vi "LABVIEWWIPPROJECT.vi"() -> ()   [LabVIEW 2025]
panel:
  out "Balance":dbl
  out "Jackpot":bool
  out "minor prize":bool
  out "String":string
  in  "Bet amount":i32
  out "Array of Nums":dbl[](array[numeric])
  out "Major Prize":bool
  in  "SPIN":bool
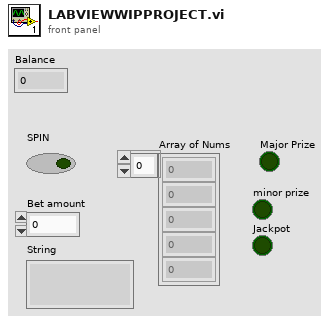
[diagram p1: front panel]
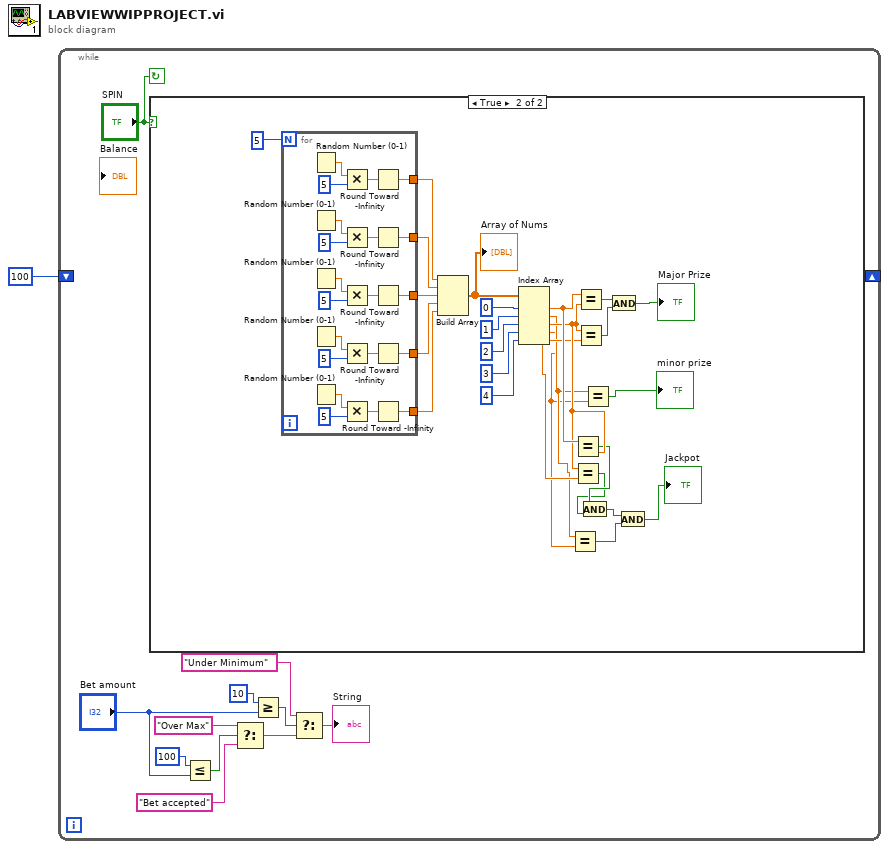
[diagram p0: block diagram]
diagram:
  n1 = while {
    shift-right: _ -> [_]
    shift-left: 100 -> [_]
    stop <- "SPIN" continue-if-true
    n2 = case shown="True" "SPIN" {
      frame False {
      }
      frame True {
        n3 = for {
          N: 5 -> [_]
          tunnel: [w43] -> w30
          tunnel: [w42] -> w29
          tunnel: [w41] -> w28
          tunnel: [w40] -> w27
          tunnel: [w39] -> w26
          n4 = Random Number (0-1)() -> (number: 0 to 1=w58:dbl)
          n5 = Random Number (0-1)() -> (number: 0 to 1=w55:dbl)
          n6 = Random Number (0-1)() -> (number: 0 to 1=w52:dbl)
          n7 = Random Number (0-1)() -> (number: 0 to 1=w49:dbl)
          n8 = Random Number (0-1)() -> (number: 0 to 1=w46:dbl)
          n9 = Multiply(x=w58, y=5) -> (x*y=w56:dbl)
          n10 = Multiply(x=w55, y=5) -> (x*y=w53:dbl)
          n11 = Multiply(x=w52, y=5) -> (x*y=w50:dbl)
          n12 = Multiply(x=w49, y=5) -> (x*y=w47:dbl)
          n13 = Multiply(x=w46, y=5) -> (x*y=w44:dbl)
          n14 = Round Toward -Infinity(1:w56) -> (0:w43:dbl)
          n15 = Round Toward -Infinity(1:w53) -> (0:w42:dbl)
          n16 = Round Toward -Infinity(1:w50) -> (0:w41:dbl)
          n17 = Round Toward -Infinity(1:w47) -> (0:w40:dbl)
          n18 = Round Toward -Infinity(1:w44) -> (0:w39:dbl)
        }
        n19 = Build Array(w30, w29, w28, w27, w26) -> (w25:dbl[])
        "Array of Nums" <- w25
        n20 = Index Array(array=w25, index #1=0, index #2=1, index #3=2, index #4=3, index #5=4) -> (element #1=w22:dbl, element #2=w19:dbl, element #3=w21:dbl, element #4=w18:dbl, element #5=w20:dbl)
        n21 = Equal?(x=w19, y=w18) -> (x = y?=w14:bool)
        n22 = Equal?(x=w22, y=w21) -> (x = y?=w17:bool)
        n23 = Equal?(x=w21, y=w20) -> (x = y?=w16:bool)
        n24 = Equal?(x=w22, y=w21) -> (x = y?=w37:bool)
        n25 = Equal?(x=w21, y=w20) -> (x = y?=w31:bool)
        n26 = And(x=w17, y=w16) -> (x .and. y?=w15:bool)
        n27 = Equal?(x=w19, y=w18) -> (x = y?=→"minor prize":bool)
        n28 = And(x=w37, y=w31) -> (x .and. y?=→"Major Prize":bool)
        n29 = And(x=w15, y=w14) -> (x .and. y?=→"Jackpot":bool)
      }
    }
    n30 = Less Or Equal?(x=100, y="Bet amount") -> (x <= y?=w6:bool)
    n31 = Select(t="Over Max", s=w6, f="Bet accepted") -> (s? t:f=w3:string)
    n32 = Greater Or Equal?(x=10, y="Bet amount") -> (x >= y?=w5:bool)
    n33 = Select(t="Under Minimum", s=w5, f=w3) -> (s? t:f=→"String":string)
  }
